vi "waitTarget-XY.vi"(0 ".NET Refnum in X":refnum<k24>, 5 "GetPOS X":refnum<vi>, 7 "Position X (mm)":sgl, 9 "GetPOS Y":refnum<vi>, 11 ".NET Refnum in Y":refnum<k24>) -> (4 ".NET Refnum out X":refnum<k24>, 6 "GetPOS X (mm)":dbl format="%#_6f", 8 "GetPOS Y (mm)":dbl format="%#_6f", 15 ".NET Refnum out Y":refnum<k24>)   [LabVIEW 2014]
doc: "André Romero - 2018\nandretec@ifsc.usp.br"
uses:
  C:/users-lab/Andre/GITs/andretec/Thorlabs-Vector-Move/kinesisTec/Kinesis/Thorlabs.MotionControl.TCube.DCServoCLI.dll
  Kinesis/Thorlabs.MotionControl.TCube.DCServoCLI.dll
panel:
  in  "Position Y (mm)":sgl
  in  "error":dbl=0.004 format="%#_13g"
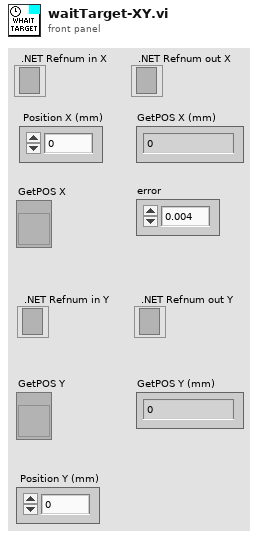
[diagram p1: front panel]
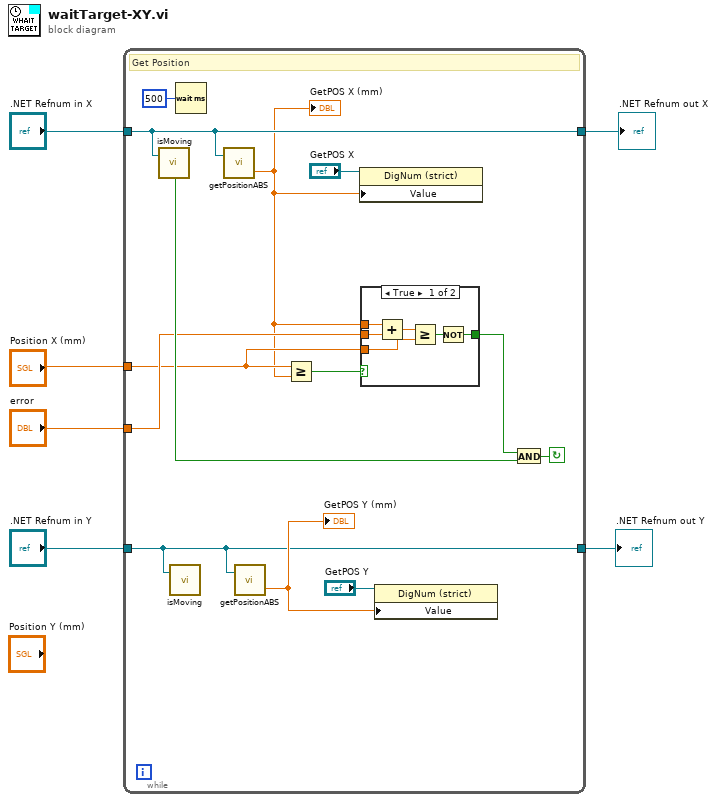
[diagram p0: block diagram]
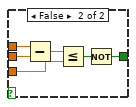
[diagram p2: hidden frame]
diagram:
  n1 = while {
    tunnel: ".NET Refnum in X" -> [w19]
    tunnel: [w19] -> w5
    tunnel: "Position X (mm)" -> [w12]
    tunnel: "error" -> [w13]
    tunnel: ".NET Refnum in Y" -> [w7]
    tunnel: [w7] -> w1
    stop <- w16 continue-if-true
    # "Get Position"
    n2 = call "isMoving.vi"("Device in"=w19) -> ("IsMoving"=w17:bool)  [unwired: 2 in]
    n3 = call "isMoving.vi"("Device in"=w7) -> ()  [unwired: 2 in, 1 out]
    n4 = Wait (ms)(milliseconds to wait=u32 500) -> ()  [unwired: 1 out]
    n5 = call "getPositionABS.vi"("Device"=w19) -> ("GetPOS"=w10:dbl)  [unwired: 1 in, 1 out]
    "GetPOS X (mm)" <- w10
    n6 = call "getPositionABS.vi"("Device"=w7) -> ("GetPOS"=w8:dbl)  [unwired: 1 in, 1 out]
    "GetPOS Y (mm)" <- w8
    n7 = Greater Or Equal?(x=w12, y=w10) -> (x >= y?=w14:bool)
    n8 = property class="DigNum (strict)"(reference="GetPOS X", "Value"=w10) -> ()  [unwired: 1 in, 2 out]
    n9 = case shown="True" w14 {
      tunnel: w10 -> [w25 w31]
      tunnel: w13 -> [w24 w30]
      tunnel: w12 -> [w22 w28]
      tunnel: [w20 w26] -> w11
      frame True {
        n10 = Add(x=w25, y=w24) -> (x+y=w23:dbl)
        n11 = Greater Or Equal?(x=w23, y=w22) -> (x >= y?=w21:bool)
        n12 = Not(x=w21) -> (.not. x?=w20:bool)
      }
      frame False {
        n13 = Subtract(x=w31, y=w30) -> (x-y=w29:dbl)
        n14 = Less Or Equal?(x=w29, y=w28) -> (x <= y?=w27:bool)
        n15 = Not(x=w27) -> (.not. x?=w26:bool)
      }
    }
    n16 = property class="DigNum (strict)"(reference="GetPOS Y", "Value"=w8) -> ()  [unwired: 1 in, 2 out]
    n17 = And(x=w11, y=w17) -> (x .and. y?=w16:bool)
  }
  ".NET Refnum out X" <- w5
  ".NET Refnum out Y" <- w1
